vi "Destructor.vi"(8 "error in":errorcluster, 11 "DateTimeMeasure":refnum<class "DateTimeMeasure.lvclass">) -> (0 "error out":errorcluster)   [LabVIEW 2021, in "ProligentXMLGenerator.lvlib" / "DateTimeMeasure.lvclass"]
uses:
  DateTimeMeasure.lvclass
  DateTimeMeasure.lvclass/DateTimeMeasure.ctl
  Measure/Measure.lvclass
  MeasureLimit/MeasureLimit.lvclass
  DateTimeMeasureLimit/DateTimeMeasureLimit.lvclass
  C:/Projects/proligent-xml-generator-labview/src/ProligentXMLGenerator/Measure/Measure/Measure.lvclass
  C:/Projects/proligent-xml-generator-labview/src/ProligentXMLGenerator/Measure/DateTimeMeasure/DateTimeMeasure.lvclass
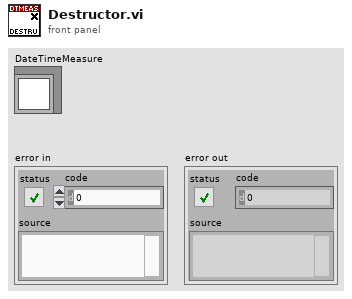
[diagram p1: front panel]
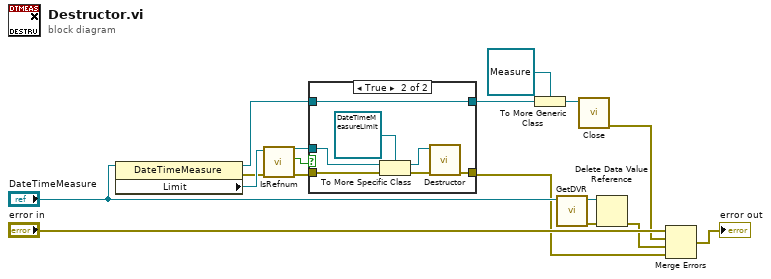
[diagram p0: block diagram]
diagram:
  n1 = property class="DateTimeMeasure"(reference="DateTimeMeasure") -> (reference out=w5:refnum<class "DateTimeMeasure.lvclass">, error out=w7:errorcluster, "Limit"=w8:refnum<class "MeasureLimit.lvclass">)  [unwired: 1 in]
  n2 = call "IsRefnum.vi"("error in"=w7, "MeasureLimit in"=w8) -> ("error out"=w11:errorcluster, "IsRefnum"=w9:bool, "MeasureLimit out"=w10:refnum<class "MeasureLimit.lvclass">)  [unwired: 7 in]
  n3 = case shown="True" w9 {
    tunnel: w11 -> [w19 w25]
    tunnel: w10 -> [_ w24]
    tunnel: [w19 w22] -> w3
    tunnel: [w18 w26] -> w6
    tunnel: w5 -> [w18 w26]
    frame False {
    }
    frame True {
      n4 = To More Specific Class(target class=refnum<class "DateTimeMeasureLimit.lvclass"> refnum ("ProligentResultProcessor:DateTimeMeasureLimit"), reference=w24, error in=w25) -> (specific class reference=w21:refnum<class "DateTimeMeasureLimit.lvclass">, error out=w23:errorcluster)
      n5 = call "Destructor.vi"("error in"=w23, "DateTimeMeasureLimit"=w21) -> ("error out"=w22:errorcluster)  [unwired: 9 in]
    }
  }
  n6 = To More Generic Class(target class=refnum<class "Measure.lvclass"> refnum ("ProligentResultProcessor:Measure"), reference=w6) -> (generic class reference=w4:refnum<class "Measure.lvclass">)
  n7 = call "GetDVR.vi"("DateTimeMeasure"="DateTimeMeasure") -> ("error out"=w15:errorcluster, "DVRReference"=w1:refnum<data-value>)  [unwired: 9 in]
  n8 = call "Close.vi"("Measure"=w4) -> ("error out"=w2:errorcluster)  [unwired: 10 in]
  n9 = Delete Data Value Reference(data value reference=w1, error in=w15) -> (error out=w14:errorcluster)  [unwired: 1 out]
  n10 = Merge Errors("error in", w2, w14, w3) -> (→"error out":errorcluster)
